vi "IMAQ-GetLineContrast.vi"(4 "Image Device":cluster{"Image":T1, "errorImage":errorcluster}, 5 "Nueva Linea?":bool) -> (0 "Gray Level Intensities":T2 {"Standard  Deviation" format="%.2f"; "Mean Intensity" format="%.2f"; "Maximum Intensity" format="%.2f"; "Minimum Intensity" format="%.2f"}, 1 "Contraste":dbl, 2 "Line Profile":dbl[](graph))   [LabVIEW 2010]
uses:
  <vilib>/vision/Image Controls.llb/IMAQ Image.ctl
  <vilib>/vision/NI_Vision_Development_Module.lvlib
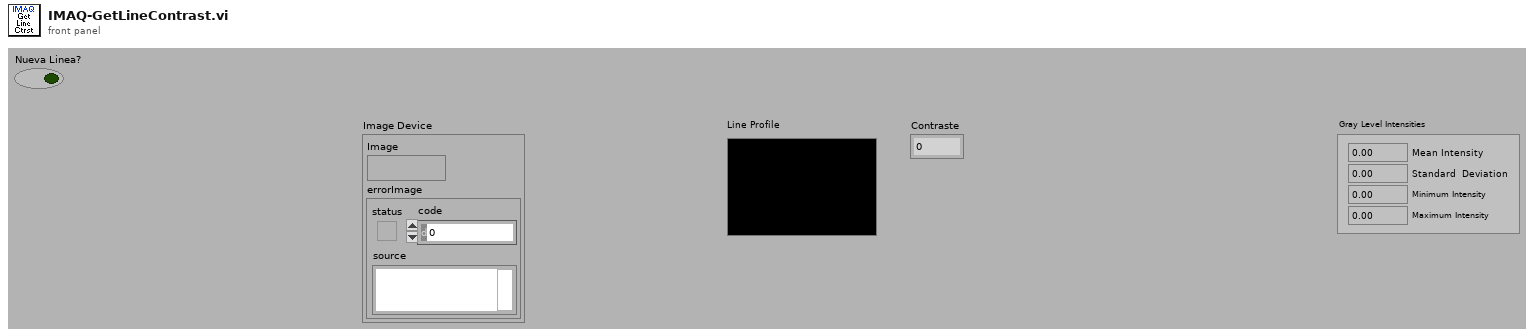
[diagram p1: front panel]
types:
  T1 = typedef "IMAQ Image.ctl" = refnum<image>
  T2 = cluster{"Mean Intensity":sgl, "Standard  Deviation":sgl, "Minimum Intensity":sgl, "Maximum Intensity":sgl}
  T3 = typedef "IMAQ Line" = cluster{"Start X":i32, "Start Y":i32, "End X":i32, "End Y":i32}
  T4 = typedef "Image Type" = u32
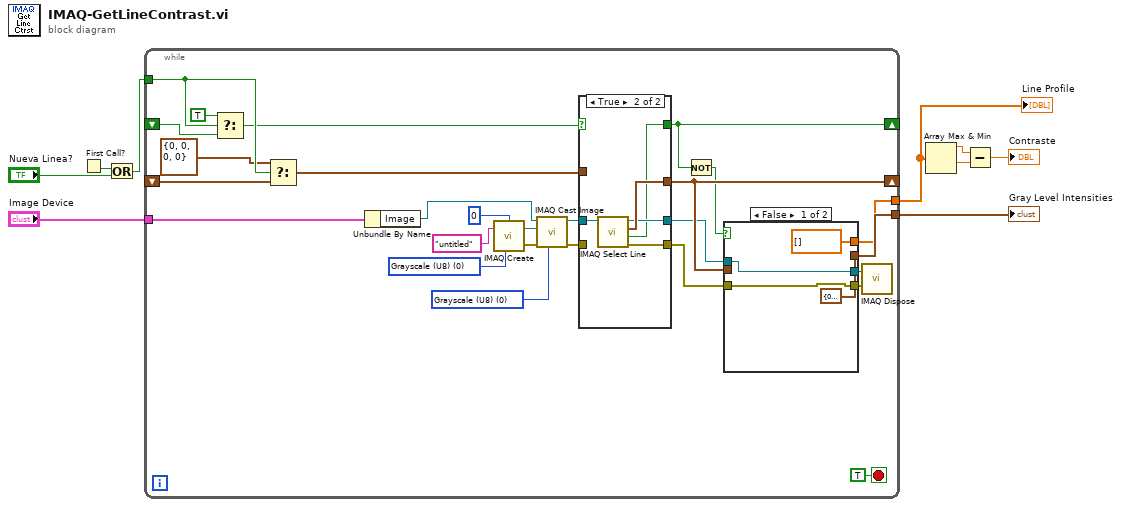
[diagram p0: block diagram]
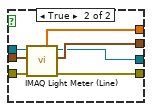
[diagram p2: hidden frame]
diagram:
  n1 = First Call?() -> (First Call?: T/F=w3:bool)
  n2 = Or(x=w3, y="Nueva Linea?") -> (x .or. y?=w4:bool)
  n3 = while {
    shift-right: [w34] -> _
    shift-left: _ -> [w17]
    tunnel: "Image Device" -> [w33]
    tunnel: [w32] -> w8
    tunnel: [w31] -> w1
    shift-right: [w12] -> _
    shift-left: _ -> [w30]
    tunnel: w4 -> [w18]
    stop <- TRUE stop-if-true
    w19 = T4 0 items=["Grayscale (U8)", "Grayscale (I16)", "Grayscale (SGL)", "Complex (CSG)", "RGB (U32)", "HSL (U32)", "RGB (U64)", "Grayscale (U16)"] ("Image Type")
    w22 = T4 0 items=["Grayscale (U8)", "Grayscale (I16)", "Grayscale (SGL)", "Complex (CSG)", "RGB (U32)", "HSL (U32)", "RGB (U64)", "Grayscale (U16)"] ("Image Type")
    n4 = Select(t=TRUE, s=w18, f=w30) -> (s? t:f=w14:bool)
    n5 = Select(t=T3 {"Start X"=0, "Start Y"=0, "End X"=0, "End Y"=0} ("Line"), s=w18, f=w17) -> (s? t:f=w15:T3)
    n6 = Unbundle By Name(w33) -> ("Image"=w36:T1)
    n7 = call "IMAQ Create"("Border Size"=0, "Image Name"="untitled", "Image Type"=w22) -> ("New Image"=w25:T1, "error out"=w20:errorcluster)  [unwired: 2 in]
    n8 = call "IMAQ Cast Image"("Image Type"=w19, "error in (no error)"=w20, "Image Dst"=w25, "Image Src"=w36) -> ("error out"=w21:errorcluster, "Image Dst Out"=w28:T1)  [unwired: 6 in]
    n9 = case shown="True" w14 {
      selector: w14 -> [w48 _]
      tunnel: w28 -> [w51 w56]
      tunnel: [w50 w55] -> w27
      tunnel: [w49 w54] -> w34
      tunnel: [w51 w53] -> w26
      tunnel: w21 -> [w50 _]
      tunnel: w15 -> [w49 _]
      tunnel: [w48 w52] -> w12
      frame False {
      }
      frame True {
        n10 = call "IMAQ Select Line"("Image In"=w56) -> ("error out"=w55:errorcluster, "Cancelled"=w52:bool, "Line"=w54:T3, "Image Out (duplicate)"=w53:T1)  [unwired: 7 in]
      }
    }
    n11 = Not(x=w12) -> (.not. x?=w13:bool)
    n12 = case shown="False" w13 {
      tunnel: w34 -> [_ w47]
      tunnel: [T2 {"Mean Intensity"=0.0, "Standard  Deviation"=0.0, "Minimum Intensity"=0.0, "Maximum Intensity"=0.0} ("Gray Level Intensities") w46] -> w32
      tunnel: [dbl[] [] ("Line Profile") w45] -> w31
      tunnel: w27 -> [w37 w44]
      tunnel: w26 -> [w38 w43]
      tunnel: [w38 w42] -> w11
      tunnel: [w37 w41] -> w10
      frame False {
      }
      frame True {
        n13 = call "IMAQ Light Meter (Line)"("error in (no error)"=w44, "Line"=w47, "Image"=w43) -> ("error out"=w41:errorcluster, "Gray Level Intensities"=w46:T2, "Image Out"=w42:T1, "Line Profile"=w45:dbl[])  [unwired: 4 in, 1 out]
      }
    }
    n14 = call "IMAQ Dispose"("Image"=w11, "error in (no error)"=w10) -> ()  [unwired: 4 in, 1 out]
  }
  "Gray Level Intensities" <- w8
  "Line Profile" <- w1
  n15 = Array Max & Min(array=w1) -> (max value=w5:dbl, min value=w6:dbl)  [unwired: 2 out]
  n16 = Subtract(x=w5, y=w6) -> (x-y=→"Contraste":dbl)
